vi "Pockels-Adjust with Z.vi"(9 "Motor Z Planes(um)":dbl[](array[numeric])=[200.0, 150.0, 100.0, 50.0, 0.0, -50.0, -100.0, -150.0, -200.0]) -> (1 "Ls (Scattering Parameter)":dbl=100.0, 3 "Laser power % corrected for depth":dbl[](array[numeric]))   [LabVIEW 2017]
panel:
  in  "Enable\nTest Input":bool
  in  "TEST INPUT":T1={"ZStack"={"Zstart"=200.0, "Zstop"=-200.0, "Zstep"=50.0}, "Laser Power %"={"@ Start"=10.0, "@ Stop"=80.0}}
  out "Waveform Graph":dbl[][](graph)
  out "Laser Power %.@ Stop":dbl
  out "Laser Power %.@ Start":dbl
  out "VI exec. time (ms)":u32
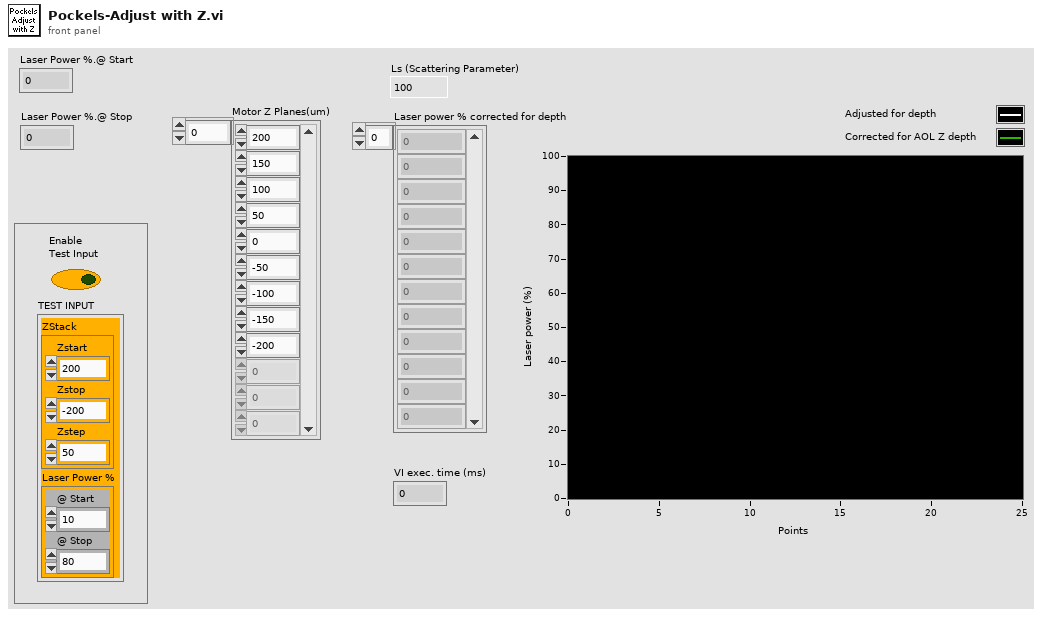
[diagram p1: front panel]
types:
  T1 = cluster{"ZStack":cluster{"Zstart":dbl, "Zstop":dbl, "Zstep":dbl}, "Laser Power %":cluster{"@ Start":dbl, "@ Stop":dbl}}
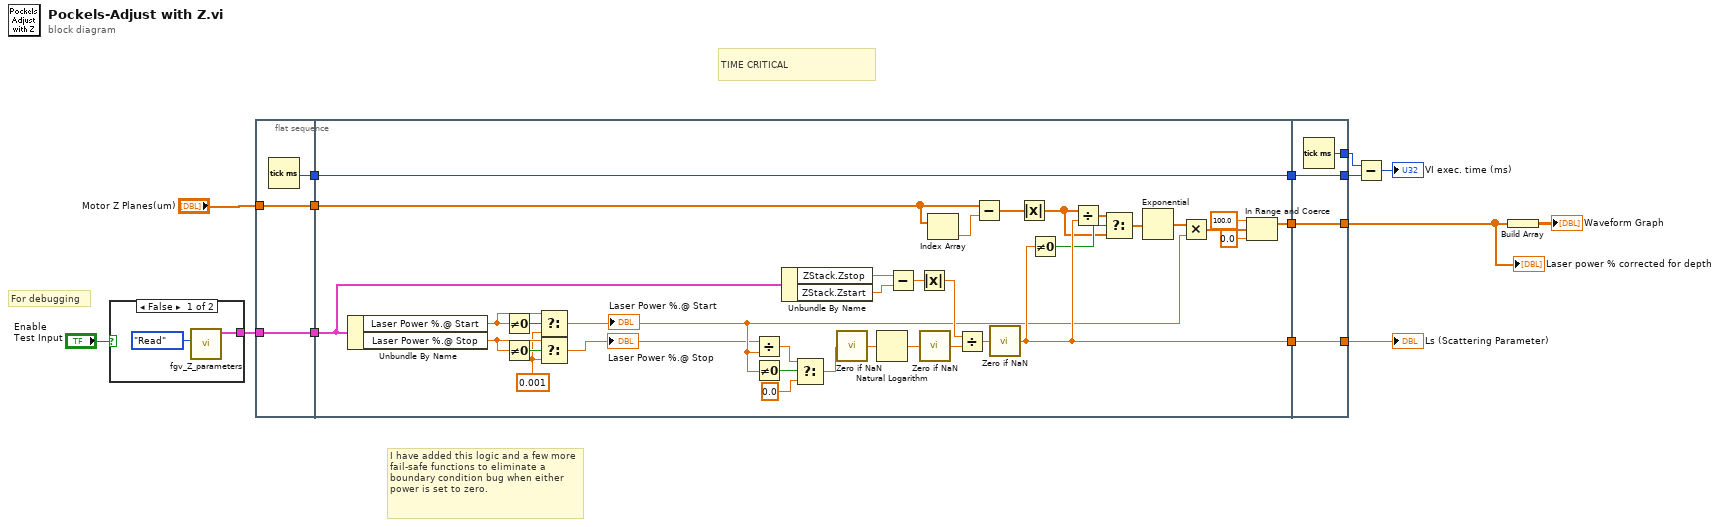
[diagram p0: block diagram]
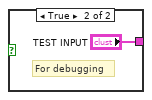
[diagram p2: hidden frame]
diagram:
  # "TIME CRITICAL"
  # "For debugging"
  # "I have added this logic and a few more fail-safe functions to eliminate a boundary condition bug when either power is set to zero."
  n1 = case shown="False" "Enable\nTest Input" {
    tunnel: [w17 "TEST INPUT"] -> w6
    frame False {
      n2 = call "fgv_Z_parameters.vi"("Function"=enum16{"Intialize", "Write", "Read", "Clear"}."Read") -> ("Z Parameters"=w17:T1)  [unwired: 9 in, 1 out]
    }
    frame True {
      # "For debugging"
    }
  }
  n3 = flat-sequence {
    tunnel: "Motor Z Planes(um)" -> [w20]
    tunnel: w6 -> [w21]
    tunnel: [w21] -> w13
    tunnel: [w20] -> w12
    tunnel: [w19] -> w10
    tunnel: [w46] -> w14
    tunnel: w13 -> [w38]
    tunnel: w12 -> [w52]
    tunnel: w10 -> [w50]
    tunnel: [w50] -> w9
    tunnel: [w22] -> w5
    tunnel: [w58] -> w15
    tunnel: [w59] -> w3
    tunnel: w14 -> [w58]
    tunnel: [w57] -> w11
    tunnel: w9 -> [w56]
    tunnel: [w56] -> w8
    tunnel: w5 -> [w59]
    frame #0 {
      n4 = Tick Count (ms)() -> (millisecond timer value=w19:u32)
    }
    frame #1 {
      w33 = 0.001 ("f")
      n5 = Unbundle By Name(w38) -> ("Laser Power %.@ Start"=w37:dbl, "Laser Power %.@ Stop"=w34:dbl)
      n6 = Not Equal To 0?(x=w37) -> (x != 0?=w39:bool)
      n7 = Not Equal To 0?(x=w34) -> (x != 0?=w35:bool)
      n8 = Select(t=w37, s=w39, f=w33) -> (s? t:f=w36:dbl)
      "Laser Power %.@ Start" <- w36
      n9 = Select(t=w34, s=w35, f=w33) -> (s? t:f=w32:dbl)
      "Laser Power %.@ Stop" <- w32
      n10 = Divide(x=w32, y=w36) -> (x/y=w31:dbl)
      n11 = Not Equal To 0?(x=w36) -> (x != 0?=w42:bool)
      n12 = Unbundle By Name(w38) -> ("ZStack.Zstop"=w40:dbl, "ZStack.Zstart"=w41:dbl)
      n13 = Select(t=w31, s=w42, f=0.0) -> (s? t:f=w29:dbl)
      n14 = call "Zero if NaN.vi"("Number In"=w29) -> ("Number Out"=w43:dbl)
      n15 = Natural Logarithm(1:w43) -> (0:w49:dbl)
      n16 = Subtract(x=w40, y=w41) -> (x-y=w54:dbl)
      n17 = Absolute Value(x=w54) -> (abs(x)=w55:dbl)
      n18 = call "Zero if NaN.vi"("Number In"=w49) -> ("Number Out"=w48:dbl)
      n19 = Index Array(array=w52) -> (element=w53:dbl)  [unwired: 1 in]
      n20 = Divide(x=w55, y=w48) -> (x/y=w47:dbl)
      n21 = Subtract(x=w52, y=w53) -> (x-y=w51:dbl[])
      n22 = call "Zero if NaN.vi"("Number In"=w47) -> ("Number Out"=w46:dbl)
      n23 = Absolute Value(x=w51) -> (abs(x)=w28:dbl[])
      n24 = Not Equal To 0?(x=w46) -> (x != 0?=w44:bool)
      n25 = Divide(x=w28, y=w46) -> (x/y=w27:dbl[])
      n26 = Select(t=w27, s=w44, f=w28) -> (s? t:f=w45:dbl[])
      n27 = Exponential(1:w45) -> (0:w26:dbl[])
      n28 = Multiply(x=w26, y=w36) -> (x*y=w23:dbl[])
      n29 = In Range and Coerce(upper limit=100.0, x=w23, lower limit=0.0) -> (coerced(x)=w22:dbl[])  [unwired: 1 out]
    }
    frame #2 {
      n30 = Tick Count (ms)() -> (millisecond timer value=w57:u32)
    }
  }
  n31 = Subtract(x=w11, y=w8) -> (x-y=→"VI exec. time (ms)":u32)
  n32 = Build Array(w3) -> (→"Waveform Graph":dbl[][])
  "Ls (Scattering Parameter)" <- w15
  "Laser power % corrected for depth" <- w3
